vi "accumulate.vi"(8 "error in (no error)":errorcluster, 11 "dataTA in":refnum<class "dataTA.lvclass">) -> (0 "error out":errorcluster, 3 "dataTA out":refnum<class "dataTA.lvclass">)   [LabVIEW 2019, in "dataTA.lvlib" / "dataTA.lvclass"]
uses:
  dataTA.lvclass
  dataTA.lvclass/dataTA.ctl
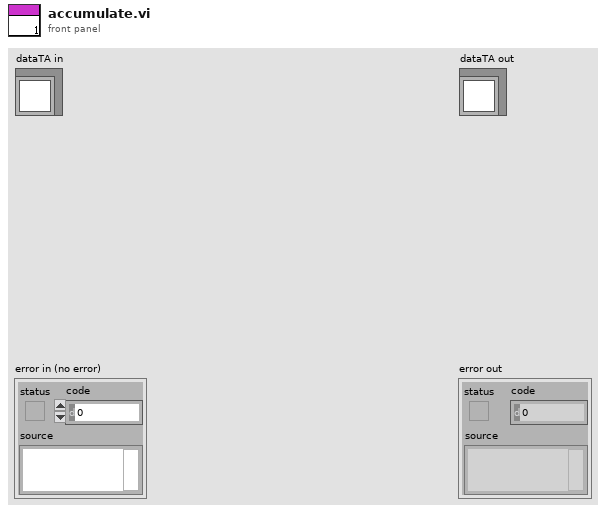
[diagram p1: front panel]
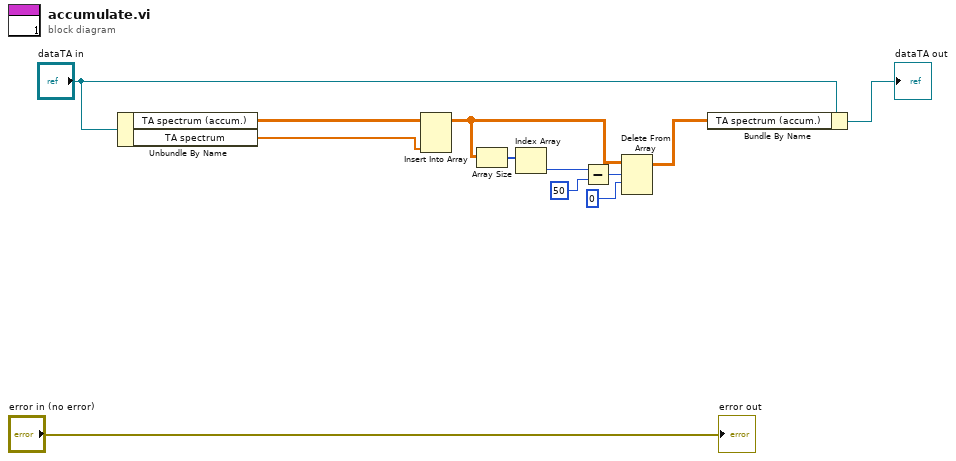
[diagram p0: block diagram]
diagram:
  n1 = Unbundle By Name("dataTA in") -> ("TA spectrum (accum.)"=w9:dbl[][], "TA spectrum"=w8:dbl[])
  n2 = Insert Into Array(array=w9, new element=w8) -> (w7:dbl[][])  [unwired: 2 in]
  n3 = Array Size(array=w7) -> (size(s)=w6:i32[])
  n4 = Index Array(array=w6) -> (element=w5:i32)  [unwired: 1 in]
  n5 = Subtract(x=w5, y=50) -> (x-y=w2:i32)
  n6 = Delete From Array(array=w7, length=w2, index (row)=0 ("length")) -> (array with subset deleted=w3:dbl[][])  [unwired: 1 in, 1 out]
  n7 = Bundle By Name(cluster="dataTA in", "TA spectrum (accum.)"=w3) -> (→"dataTA out":refnum<class "dataTA.lvclass">)
  "error out" <- "error in (no error)"
